vi "p2.vi"() -> ()   [LabVIEW 2023, in "d17.lvlib"]
uses:
  d17.lvlib
  AOC/AOC.lvlib
panel:
  out "min value":u64
  in  "Example":string="2413432311323\n3215453535623\n3255245654254\n3446585845452\n4546657867536\n1438598798454\n4457876987766\n3637877979653\n4654967986887\n4564679986453\n1224686865563\n2546548887735\n4322674655533"
  in  "Example":bool
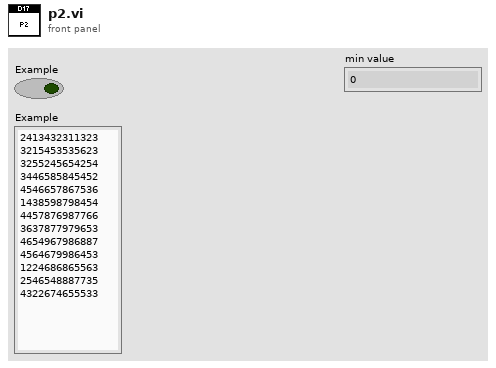
[diagram p1: front panel]
types:
  T1 = map{cluster{"unsigned 8bit integer":i16, "unsigned 8bit integer":i16}, cluster{"unsigned 8bit integer":i16, "unsigned 8bit integer":i16}[]}
  T2 = cluster{"heat loss":u64, "position":cluster{"unsigned 8bit integer":i16, "unsigned 8bit integer":i16}, "direction":cluster{"unsigned 8bit integer":i16, "unsigned 8bit integer":i16}}
  T3 = cluster{"unsigned 8bit integer":i16, "unsigned 8bit integer":i16}
  T4 = map{cluster{cluster{"unsigned 8bit integer":i16, "unsigned 8bit integer":i16}, "RIGHT":cluster{"unsigned 8bit integer":i16, "unsigned 8bit integer":i16}}, u64}
  T5 = cluster{cluster{"unsigned 8bit integer":i16, "unsigned 8bit integer":i16}, "RIGHT":cluster{"unsigned 8bit integer":i16, "unsigned 8bit integer":i16}}
  T6 = cluster{cluster{"unsigned 8bit integer":i16, "unsigned 8bit integer":i16}, "LEFT":cluster{"unsigned 8bit integer":i16, "unsigned 8bit integer":i16}}
  T7 = cluster{cluster{"unsigned 8bit integer":i16, "unsigned 8bit integer":i16}, "UP":cluster{"unsigned 8bit integer":i16, "unsigned 8bit integer":i16}}
  T8 = cluster{cluster{"unsigned 8bit integer":i16, "unsigned 8bit integer":i16}, "DOWN":cluster{"unsigned 8bit integer":i16, "unsigned 8bit integer":i16}}
  T9 = cluster{cluster{"unsigned 8bit integer":i16, "unsigned 8bit integer":i16}, "DOWN":cluster{"unsigned 8bit integer":i16, "unsigned 8bit integer":i16}}[]
  T10 = cluster{"unsigned 8bit integer":i16, "unsigned 8bit integer":i16}[]
  T11 = cluster{"position":cluster{"unsigned 8bit integer":i16, "unsigned 8bit integer":i16}, "direction":cluster{"unsigned 8bit integer":i16, "unsigned 8bit integer":i16}}
  T12 = cluster{u64, cluster{"unsigned 8bit integer":i16, "unsigned 8bit integer":i16}, "RIGHT":cluster{"unsigned 8bit integer":i16, "unsigned 8bit integer":i16}}
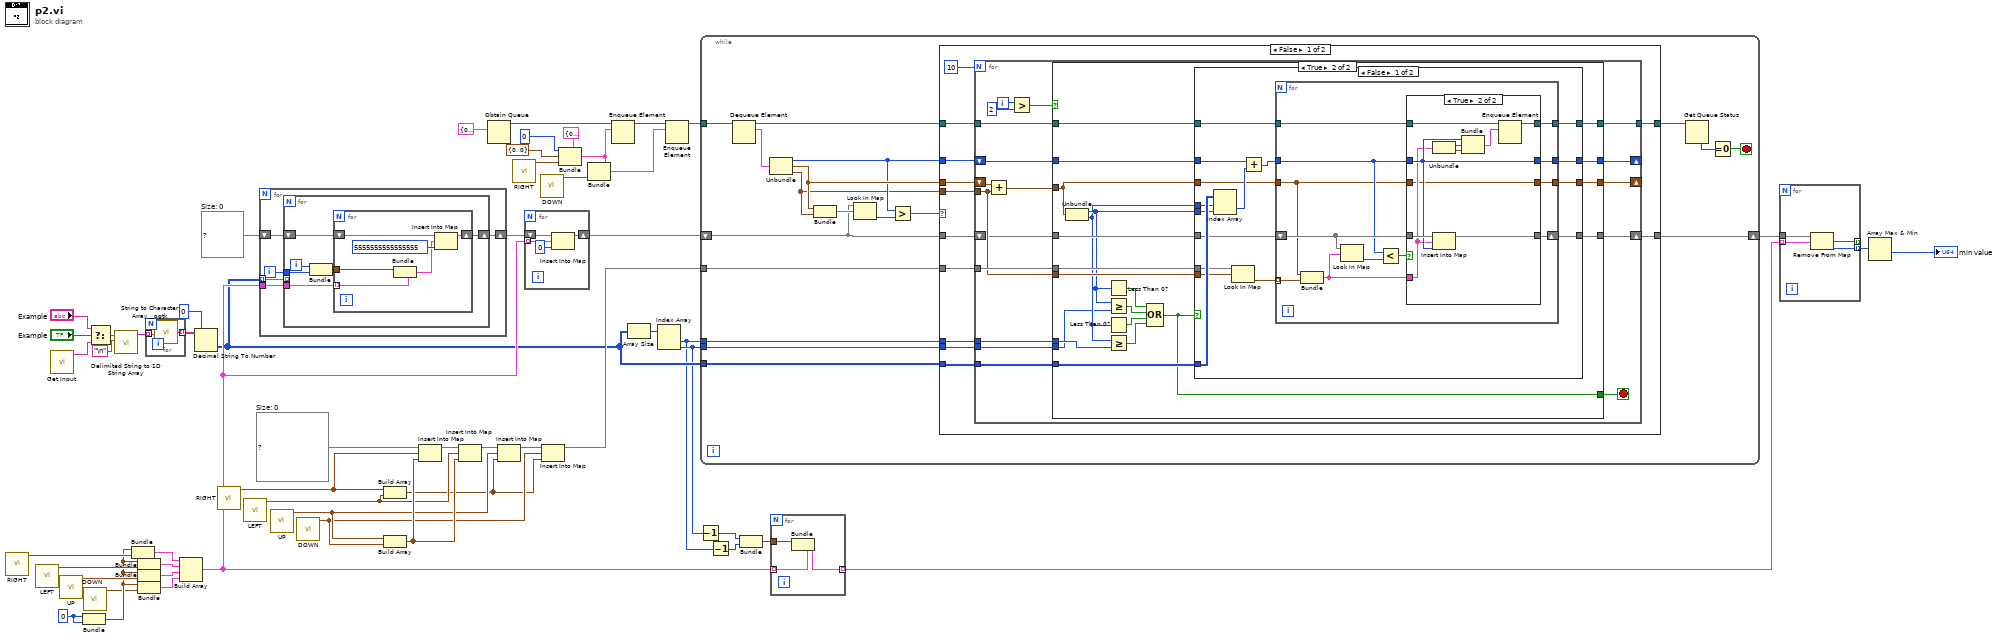
[diagram p0: block diagram]
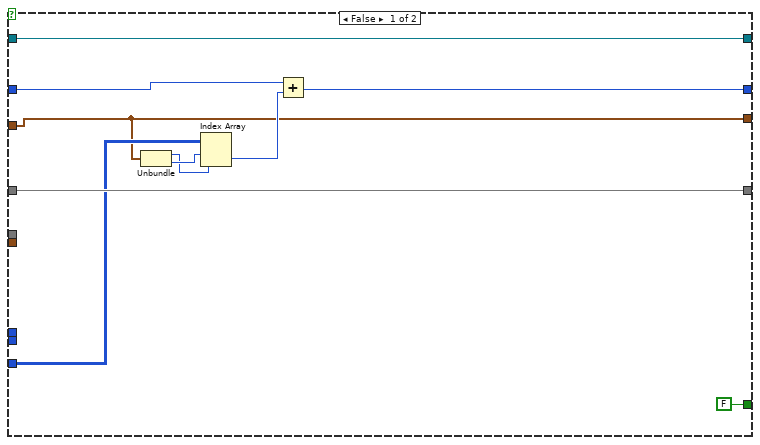
[diagram p2: hidden frame]
diagram:
  w34 = T1 {}  # Size: 0
  w52 = i16 0 ("unsigned 8bit integer")
  w19 = T4 {}  # Size: 0
  n1 = call "RIGHT.vi"() -> ("RIGHT"=w51:T3)  [unwired: 11 in]
  n2 = call "LEFT.vi"() -> ("LEFT"=w50:T3)  [unwired: 11 in]
  n3 = call "Get Input.vi"() -> ("Input"=w55:string)  [unwired: 11 in]
  n4 = call "UP.vi"() -> ("UP"=w49:T3)  [unwired: 11 in]
  n5 = Bundle("unsigned 8bit integer"=w52, "unsigned 8bit integer"=w52) -> (w48:T3)  [unwired: 1 in]
  n6 = call "DOWN.vi"() -> ("DOWN"=w47:T3)  [unwired: 11 in]
  n7 = Select(t="Example", s="Example", f=w55) -> (s? t:f=w13:string)
  n8 = call <vilib>:"Delimited String to 1D String Array.vi"("delimiter"="\n", "delimited string"=w13) -> ("string array"=w10:string[])  [unwired: 9 in]
  n9 = Bundle(w48, "RIGHT"=w51) -> (w18:T5)  [unwired: 1 in]
  n10 = Bundle(w48, "LEFT"=w50) -> (w17:T6)  [unwired: 1 in]
  n11 = Bundle(w48, "UP"=w49) -> (w16:T7)  [unwired: 1 in]
  n12 = Bundle(w48, "DOWN"=w47) -> (w15:T8)  [unwired: 1 in]
  n13 = for {
    tunnel: w10 -> [w57] mode=indexing
    tunnel: [w56] -> w11 mode=indexing
    n14 = call <userlib>:"String to Character Array__ogtk.vi"("Input String"=w57) -> ("Character Array"=w56:string[])
  }
  n15 = Build Array(w18, w17, w16, w15) -> (w6:T9)
  n16 = Decimal String To Number(string=w11, default (0L)=u64 0 ("default (0 I32)")) -> (number=w4:u64[][])  [unwired: 1 in, 1 out]
  n17 = call "RIGHT.vi"() -> ("RIGHT"=w30:T3)  [unwired: 11 in]
  n18 = call "LEFT.vi"() -> ("LEFT"=w29:T3)  [unwired: 11 in]
  n19 = for {
    shift-right: [w60] -> w14
    shift-left: w19 -> [w62]
    tunnel: w4 -> [w58] mode=indexing
    tunnel: w6 -> [w59]
    i -> [w61]
    n20 = for {
      shift-right: [w66] -> w60
      shift-left: w62 -> [w65]
      tunnel: w61 -> [w67]
      tunnel: w59 -> [w64]
      tunnel: w58 -> [_] mode=indexing
      i -> [w68]
      n21 = Bundle(w68, w67) -> (w63:cluster{i32, i32})  [unwired: 1 in]
      n22 = for {
        tunnel: w64 -> [w73] mode=indexing
        shift-right: [w74] -> w66
        shift-left: w65 -> [w72]
        tunnel: w63 -> [w69]
        n23 = Bundle(cluster=w73, w69) -> (w70:T8)  [unwired: 1 in]
        n24 = Insert Into Map(map in=w72, key=w70, value=u64 5555555555555555) -> (map out=w74:T4)  [unwired: 2 out]
      }
    }
  }
  n25 = call "UP.vi"() -> ("UP"=w28:T3)  [unwired: 11 in]
  n26 = call "DOWN.vi"() -> ("DOWN"=w26:T3)  [unwired: 11 in]
  n27 = Build Array(w30, w29) -> (w25:T10)
  n28 = Build Array(w28, w26) -> (w32:T10)
  n29 = Insert Into Map(map in=w34, key=w30, value=w32) -> (map out=w33:T1)  [unwired: 2 out]
  n30 = Insert Into Map(map in=w33, key=w29, value=w32) -> (map out=w31:T1)  [unwired: 2 out]
  n31 = Obtain Queue(element data type=T2 {"heat loss"=0, "position"={"unsigned 8bit integer"=0, "unsigned 8bit integer"=0}, "direction"={"unsigned 8bit integer"=0, "unsigned 8bit integer"=0}} ("cluster")) -> (queue out=w41:refnum<queue>)  [unwired: 4 in, 2 out]
  n32 = Insert Into Map(map in=w31, key=w28, value=w25) -> (map out=w27:T1)  [unwired: 2 out]
  n33 = call "RIGHT.vi"() -> ("RIGHT"=w46:T3)  [unwired: 11 in]
  n34 = for {
    tunnel: w6 -> [w77] mode=indexing
    shift-right: [w78] -> w5
    shift-left: w14 -> [w76]
    n35 = Insert Into Map(map in=w76, key=w77, value=u64 0) -> (map out=w78:T4)  [unwired: 2 out]
  }
  n36 = call "DOWN.vi"() -> ("DOWN"=w39:T3)  [unwired: 11 in]
  n37 = Insert Into Map(map in=w27, key=w26, value=w25) -> (map out=w24:T1)  [unwired: 2 out]
  n38 = Bundle(cluster=T2 {"heat loss"=0, "position"={"unsigned 8bit integer"=0, "unsigned 8bit integer"=0}, "direction"={"unsigned 8bit integer"=0, "unsigned 8bit integer"=0}}, "heat loss"=u64 0 ("value"), "position"=T3 {"unsigned 8bit integer"=0, "unsigned 8bit integer"=0} ("output cluster"), "direction"=w46) -> (w40:T2)
  n39 = Bundle(cluster=w40, "direction"=w39) -> (w38:T2)  [unwired: 2 in]
  n40 = Enqueue Element(queue=w41, element=w40) -> (queue out=w37:refnum<queue>)  [unwired: 2 in, 2 out]
  n41 = Array Size(array=w4) -> (size(s)=w35:i32[])
  n42 = Index Array(array=w35) -> (element #1=w1:i32, element #2=w2:i32)  [unwired: 2 in]
  n43 = Enqueue Element(queue=w37, element=w38) -> (queue out=w36:refnum<queue>)  [unwired: 2 in, 2 out]
  n44 = Decrement(x=w2) -> (x-1=w23:i32)
  n45 = while {
    tunnel: w36 -> [w94]
    tunnel: w1 -> [w89]
    tunnel: w2 -> [w88]
    tunnel: w4 -> [w87]
    tunnel: w24 -> [w84]
    shift-right: [w82] -> w3
    shift-left: w5 -> [w83]
    stop <- w95 stop-if-true
    n46 = Dequeue Element(queue=w94) -> (queue out=w81:refnum<queue>, element=w93:T2)  [unwired: 2 in, 2 out]
    n47 = Unbundle(w93) -> ("heat loss"=w86:u64, "position"=w90:T3, "direction"=w85:T3)
    n48 = Bundle("position"=w90, "direction"=w85) -> (w92:T11)  [unwired: 1 in]
    n49 = Look In Map(map=w83, key=w92) -> (value=w91:u64)  [unwired: 1 in, 1 out]
    n50 = Greater?(x=w86, y=w91) -> (0:w79:bool)
    n51 = case shown="False" w79 {
      tunnel: w90 -> [w108 _]
      tunnel: w85 -> [w106 _]
      tunnel: w89 -> [w105 _]
      tunnel: w88 -> [w104 _]
      tunnel: w87 -> [w103 _]
      tunnel: w86 -> [w102 _]
      tunnel: w84 -> [w101 _]
      tunnel: w83 -> [w100 w204]
      tunnel: [w99 w204] -> w82
      tunnel: w81 -> [w98 w203]
      tunnel: [w97 w203] -> w80
      frame False {
        n52 = for {
          N: 10 -> [_]
          tunnel: w106 -> [w119]
          tunnel: w105 -> [w125]
          tunnel: w104 -> [w124]
          tunnel: w103 -> [w123]
          shift-right: [w121] -> _
          shift-left: w102 -> [w122]
          tunnel: w101 -> [w120]
          shift-right: [w116] -> w99
          shift-left: w100 -> [w118]
          tunnel: w98 -> [w115]
          tunnel: [w114] -> w97
          shift-right: [w113] -> _
          shift-left: w108 -> [w126]
          i -> [w112]
          stop <- w110 stop-if-true
          n53 = Add(x=w126, y=w119) -> (x+y=w117:T3)
          n54 = Greater?(x=w112, y=2) -> (0:w109:bool)
          n55 = case shown="True" w109 {
            tunnel: w125 -> [_ w138]
            tunnel: w124 -> [_ w137]
            tunnel: w123 -> [w132 w156]
            tunnel: w122 -> [w135 w155]
            tunnel: [w131 w154] -> w121
            tunnel: w120 -> [_ w153]
            tunnel: w119 -> [_ w152]
            tunnel: w118 -> [w134 w151]
            tunnel: w117 -> [w129 w150]
            tunnel: [w134 w149] -> w116
            tunnel: w115 -> [w136 w148]
            tunnel: [w136 w147] -> w114
            tunnel: [w129 w146] -> w113
            tunnel: [FALSE w145] -> w110
            frame False {
              n56 = Unbundle(w129) -> ("unsigned 8bit integer"=w127:i16, "unsigned 8bit integer"=w128:i16)
              n57 = Index Array(array=w132, index (row)=w128, index (col)=w127) -> (element=w130:u64)
              n58 = Add(x=w135, y=w130) -> (x+y=w131:u64)
            }
            frame True {
              n59 = Unbundle(w150) -> ("unsigned 8bit integer"=w140:i16, "unsigned 8bit integer"=w139:i16)
              n60 = Less Than 0?(x=w140) -> (x < 0?=w144:bool)
              n61 = Greater Or Equal?(x=w140, y=w137) -> (x >= y?=w143:bool)
              n62 = Less Than 0?(x=w139) -> (x < 0?=w142:bool)
              n63 = Greater Or Equal?(x=w139, y=w138) -> (x >= y?=w141:bool)
              n64 = Compound Arithmetic op=OR(w144, w143, w142, w141) -> (w145:bool)
              n65 = case shown="False" w145 {
                tunnel: w156 -> [w172 _]
                tunnel: w140 -> [w171 _]
                tunnel: w139 -> [w163 _]
                tunnel: w155 -> [w170 w202]
                tunnel: [w158 w202] -> w154
                tunnel: w152 -> [w168 _]
                tunnel: w153 -> [w167 _]
                tunnel: w151 -> [w164 w201]
                tunnel: w150 -> [w162 w199]
                tunnel: [w161 w201] -> w149
                tunnel: w148 -> [w160 w200]
                tunnel: [w159 w200] -> w147
                tunnel: [w157 w199] -> w146
                frame False {
                  n66 = Index Array(array=w172, index (row)=w163, index (col)=w171) -> (element=w169:u64)
                  n67 = Look In Map(map=w167, key=w168) -> (value=w166:T10)  [unwired: 1 in, 1 out]
                  n68 = Add(x=w170, y=w169) -> (x+y=w165:u64)
                  n69 = for {
                    tunnel: w166 -> [w184] mode=indexing
                    tunnel: w165 -> [w181]
                    tunnel: w162 -> [w174]
                    shift-right: [w179] -> w161
                    shift-left: w164 -> [w182]
                    tunnel: w160 -> [w178]
                    tunnel: [w177] -> w159
                    tunnel: [w176] -> w158
                    tunnel: [w173] -> w157
                    n70 = Bundle(w174, "RIGHT"=w184) -> (w180:T5)  [unwired: 1 in]
                    n71 = Look In Map(map=w182, key=w180) -> (value=w183:u64)  [unwired: 1 in, 1 out]
                    n72 = Less?(x=w181, y=w183) -> (x < y?=w175:bool)
                    n73 = case shown="True" w175 {
                      tunnel: w182 -> [w188 w198]
                      tunnel: w181 -> [w186 w194]
                      tunnel: w180 -> [_ w193]
                      tunnel: [w188 w197] -> w179
                      tunnel: w178 -> [w187 w196]
                      tunnel: [w187 w195] -> w177
                      tunnel: [w186 w194] -> w176
                      tunnel: w174 -> [w185 w189]
                      tunnel: [w185 w189] -> w173
                      frame False {
                      }
                      frame True {
                        n74 = Insert Into Map(map in=w198, key=w193, value=w194) -> (map out=w197:T4)  [unwired: 2 out]
                        n75 = Unbundle(w193) -> (w192:T3, "RIGHT"=w191:T3)
                        n76 = Bundle(w194, w192, "RIGHT"=w191) -> (w190:T12)  [unwired: 1 in]
                        n77 = Enqueue Element(queue=w196, element=w190) -> (queue out=w195:refnum<queue>)  [unwired: 2 in, 2 out]
                      }
                    }
                  }
                }
                frame True {
                }
              }
            }
          }
        }
      }
      frame True {
      }
    }
    n78 = Get Queue Status(queue=w80) -> (# elements in queue=w96:i32)  [unwired: 2 in, 7 out]
    n79 = Equal To 0?(x=w96) -> (x = 0?=w95:bool)
  }
  n80 = Decrement(x=w1) -> (x-1=w22:i32)
  n81 = Bundle(w23, w22) -> (w7:cluster{i32, i32})  [unwired: 1 in]
  n82 = for {
    tunnel: [w206] -> w8 mode=indexing
    tunnel: w6 -> [w207] mode=indexing
    tunnel: w7 -> [w205]
    n83 = Bundle(cluster=w207, w205) -> (w206:T8)  [unwired: 1 in]
  }
  n84 = for {
    tunnel: w3 -> [w211]
    tunnel: w8 -> [w210] mode=indexing
    tunnel: [w209] -> w21 mode=indexing
    tunnel: [w208] -> _ mode=indexing
    n85 = Remove From Map(10:w210, 11:w211) -> (1:w209:u64, 2:w208:bool)  [unwired: 1 out]
  }
  n86 = Array Max & Min(array=w21) -> (min value=→"min value":u64)  [unwired: 3 out]
